vi "传感器偏移.vi"() -> ()   [LabVIEW 2020]
panel:
  in  "传感器手动修正":T1
  in  "传感器偏移":T1
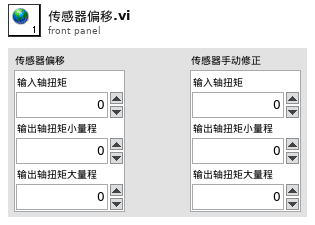
[diagram p1: front panel]
types:
  T1 = cluster{"输入轴扭矩":dbl, "输出轴扭矩小量程":dbl, "输出轴扭矩大量程":dbl}
diagram:
